vi "Global Data(冲突时的文件备份2013-03-27 14-09-21).vi"(8 "错误输入（无错误）":errorcluster, 9 "Mode":enum16{"Set", "Get", "Free"}(ring), 10 "Value In":variant, 11 "Name":string) -> (0 "错误输出":errorcluster)   [LabVIEW 2012, in "Application.lvlib"]
uses:
  Application.lvlib
panel:
  out "Value Out":variant
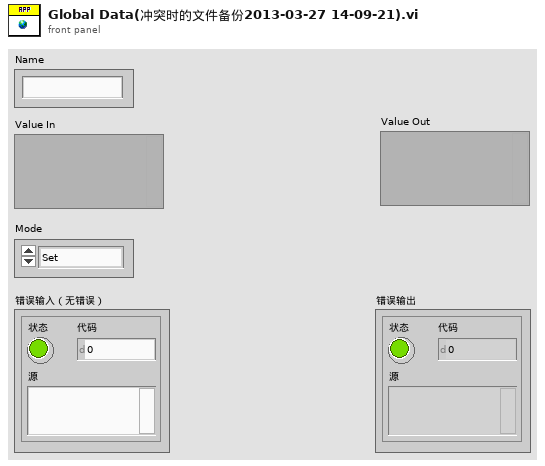
[diagram p1: front panel]
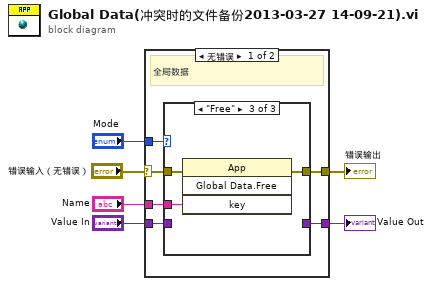
[diagram p0: block diagram]
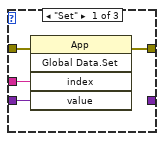
[diagram p2: hidden frame]
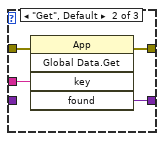
[diagram p3: hidden frame]
diagram:
  n1 = case shown="无错误" "错误输入（无错误）" {
    selector: "错误输入（无错误）" -> [w12 w24]
    tunnel: [w11 w24] -> w5
    tunnel: "Value In" -> [w10 _]
    tunnel: "Name" -> [w9 _]
    tunnel: [w8 _] -> w2
    tunnel: "Mode" -> [w7 _]
    frame No Error {
      # "全局数据"
      n2 = case shown="\"Free\"" w7 {
        tunnel: w12 -> [w16 w20 w23]
        tunnel: [w15 w19 w22] -> w11
        tunnel: w10 -> [w14 _ _]
        tunnel: w9 -> [w13 w17 w21]
        tunnel: [_ w18 _] -> w8
        frame "Set" {
          n3 = invoke class="App" method="Global Data.Set"(error in=w16, "index"=w13, "value"=w14) -> (error out=w15:errorcluster)  [unwired: 2 in, 4 out]
        }
        frame "Get", Default {
          n4 = invoke class="App" method="Global Data.Get"(error in=w20, "key"=w17) -> (error out=w19:errorcluster, "found"=w18:variant)  [unwired: 3 in, 3 out]
        }
        frame "Free" {
          n5 = invoke class="App" method="Global Data.Free"(error in=w23, "key"=w21) -> (error out=w22:errorcluster)  [unwired: 2 in, 3 out]
        }
      }
    }
    frame Error {
    }
  }
  "错误输出" <- w5
  "Value Out" <- w2
